vi "Limelight Driving Pipeline.vi"(8 "error in (no error)":errorcluster, 11 "Set Pipeline":bool) -> (0 "error out":errorcluster)   [LabVIEW 2019]
uses:
  <vilib>/Rock Robotics/Network Tables/NT Write Number.vi
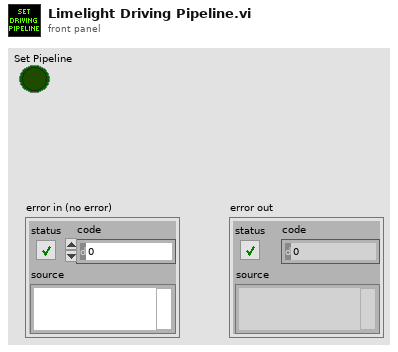
[diagram p1: front panel]
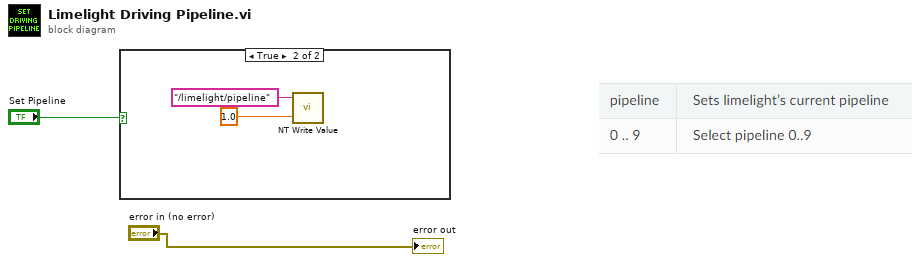
[diagram p0: block diagram]
diagram:
  n1 = case shown="True" "Set Pipeline" {
    frame False {
    }
    frame True {
      n2 = call-poly <vilib>:"NT Write Value.vi"("Numeric"=1.0, "Name"="/limelight/pipeline") -> ()  [unwired: 9 in, 1 out]
    }
  }
  "error out" <- "error in (no error)"
